vi "7_ВПСтроки.vi"() -> ()   [LabVIEW 2016]
panel:
  out "Combined String":string
  in  "Trailer":string
  in  "Header":string
  out "Length of String":dbl
  in  "Number":dbl
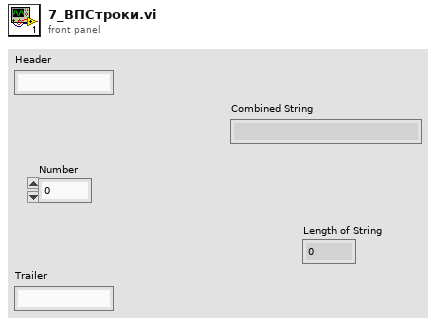
[diagram p1: front panel]
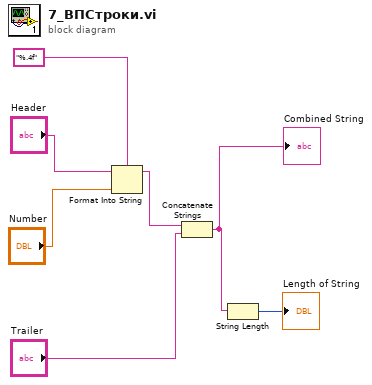
[diagram p0: block diagram]
diagram:
  n1 = Format Into String(format string="%.4f", initial string="Header", "Number") -> (resulting string=w4:string)  [unwired: 1 in, 1 out]
  n2 = Concatenate Strings(w4, "Trailer") -> (w1:string)
  "Combined String" <- w1
  n3 = String Length(string=w1) -> (length=→"Length of String":i32)
